vi "library_variable.vi"() -> ()   [LabVIEW 2020, in "queue_display_loop_1.lvlib"]
uses:
  queue_display_loop_1.lvlib
  PTRL/dev_and_debug_tools/QueueMessage typedef.ctl
  PTRL/dev_and_debug_tools/dev_and_debug_tools.lvlib
panel:
  in  "ALA_Display_Queue ref":refnum<queue>
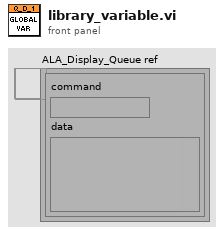
[diagram p1: front panel]
diagram:
